vi "find.vi"(11 "Array":bool[](array[boolean])) -> (3 "Index":i32)   [LabVIEW 2016]
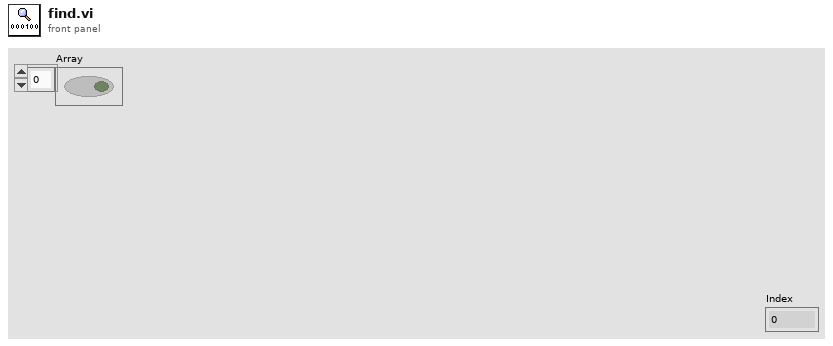
[diagram p1: front panel]
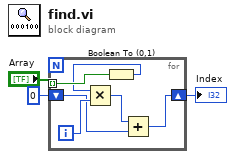
[diagram p0: block diagram]
diagram:
  n1 = for {
    tunnel: "Array" -> [w8] mode=indexing
    shift-right: [w4] -> w2
    shift-left: 0 -> [w5]
    i -> [w9]
    n2 = Boolean To (0,1)(Boolean=w8) -> (0, 1=w7:i16)
    n3 = Multiply(x=w7, y=w9) -> (x*y=w6:i32)
    n4 = Add(x=w6, y=w5) -> (x+y=w4:i32)
  }
  "Index" <- w2
